vi "Task1.vi"() -> ()   [LabVIEW 2016]
uses:
  <vilib>/NXT/Block Support/NXT_OutputPort.ctl
  <vilib>/NXT/NXTIO Xnodes/NXTIONodeSubVIs/NXTMotorRunDistance.vi
  <vilib>/NXT/NXTIO Xnodes/NXTIONodeSubVIs/NXTStopMotors.vi
  <vilib>/NXT/Dual Mode Library/Waits/Wait_Num.vi
  <vilib>/NXT/NXTIO Xnodes/AddressXNode/NXTIOAddress.xnode
  <vilib>/NXT/Subs/LVHSConnector.ctl
  <vilib>/NXT/NXTIO Xnodes/NXTIOXNode/NXTIO.xnode
  <vilib>/NXT/LegoClasses/BrickReference/BrickReference.lvclass
panel:
  in  "stop":bool
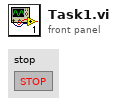
[diagram p1: front panel]
types:
  T1 = typedef "NXT_OutputPort.ctl" = u8
  T2 = typedef "LVHSConnector.ctl" = refnum<class "BrickReference.lvclass">
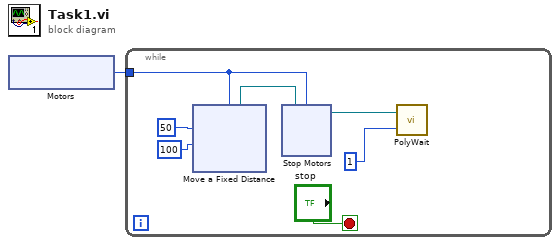
[diagram p0: block diagram]
diagram:
  n1 = xnode "Motors"() -> ("Motor"=w1:T1)
  n2 = while {
    tunnel: w1 -> [w4]
    stop <- "stop" stop-if-true
    n3 = xnode "Move a Fixed Distance"("Speed 1"=100, "Distance 1"=50, "Motors"=w4) -> ("NXT/EV3"=w7:T2)  [unwired: 1 in]
    n4 = xnode "Stop Motors"("Motors"=w4, "NXT/EV3"=w7) -> ("NXT/EV3"=w3:T2)
    n5 = call-poly <vilib>:"PolyWait.vi"("Time (1 sec)"=1, "NXT/EV3"=w3) -> ()  [unwired: 2 in, 1 out]
  }
